vi "Wait on Listener.vi"(8 "error in (no error)":errorcluster, 10 "timeout ms (wait forever: -1)":i32, 11 "TCP slave in":refnum<class "TCP Slave.lvclass">) -> (0 "error out":errorcluster, 1 "timed out?":bool, 2 "connection reference":refnum<data-value>, 3 "TCP slave out":refnum<class "TCP Slave.lvclass">)   [LabVIEW 2020, in "SubVIs.lvlib" / "TCP Slave.lvclass"]
doc: "Wrapper for the wait on listener VI, using the listener stored in the slave and an infinite timeout. When a connection is established, the output class will contain the new connection."
uses:
  <vilib>/Modbus/subvis/Protocol/TCP/TCP Slave/TCP Slave.lvclass
  <vilib>/Modbus/subvis/Protocol/TCP/TCP Slave/TCP Slave.lvclass/TCP Slave.ctl
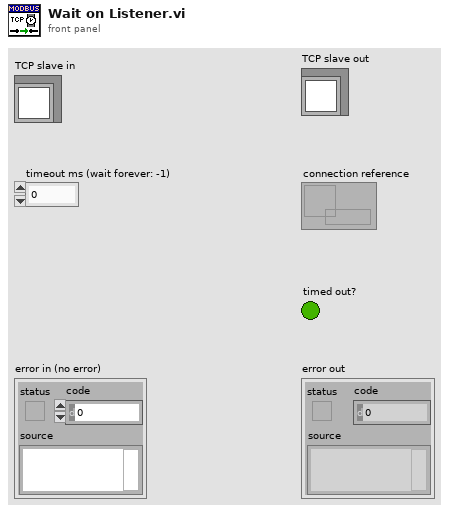
[diagram p1: front panel]
types:
  T1 = cluster{"Connected?":bool, "IP address":string, "connection error":errorcluster}
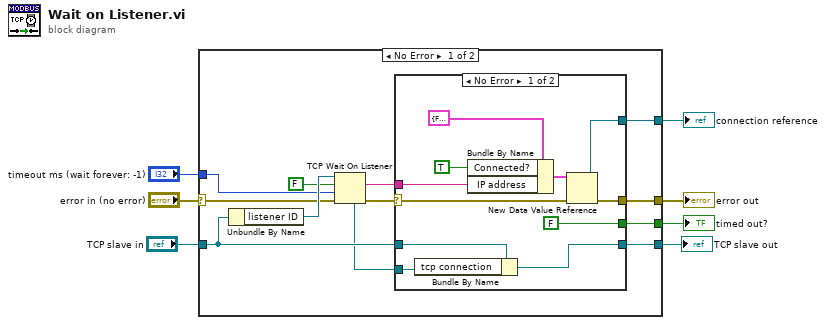
[diagram p0: block diagram]
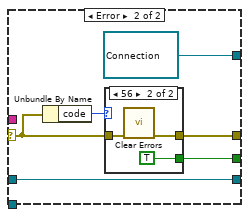
[diagram p2: hidden frame]
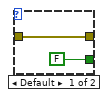
[diagram p3: hidden frame]
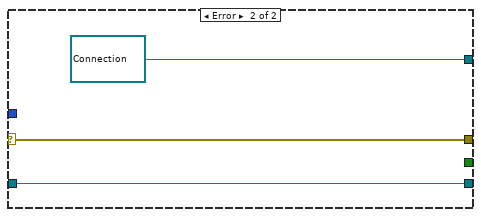
[diagram p4: hidden frame]
diagram:
  n1 = case shown="No Error" "error in (no error)" {
    selector: "error in (no error)" -> [w8 w43]
    tunnel: "TCP slave in" -> [w19 w42]
    tunnel: "timeout ms (wait forever: -1)" -> [w15 _]
    tunnel: [w14 w42] -> w5
    tunnel: [w12 w43] -> w4
    tunnel: [w11 _] -> w3
    tunnel: [w10 refnum<data-value> refnum ("data value reference")] -> w2
    frame No Error {
      n2 = Unbundle By Name(w19) -> ("listener ID"=w18:refnum<k5>)
      n3 = TCP Wait On Listener(8:w8, 9:w15, 10:FALSE ("resolve remote address (T)"), 11:w18) -> (0:w13:errorcluster, 2:w9:string, 4:w17:refnum<k5>)  [unwired: 2 out]
      n4 = case shown="No Error" w13 {
        selector: w13 -> [w26 w35]
        tunnel: w19 -> [w30 w32]
        tunnel: w17 -> [w29 _]
        tunnel: [w27 w32] -> w14
        tunnel: [w20 w34] -> w12
        tunnel: [FALSE w33] -> w11
        tunnel: [w25 refnum<data-value> refnum ("data value reference")] -> w10
        tunnel: w9 -> [w21 _]
        frame No Error {
          n5 = Bundle By Name(cluster=w30, "tcp connection"=w29) -> (w27:refnum<class "TCP Slave.lvclass">)
          n6 = Bundle By Name(cluster=T1 {"Connected?"=FALSE, "IP address"="", "connection error"={"status"=FALSE, "code"=0, "source"=""}} ("Connection"), "Connected?"=TRUE, "IP address"=w21) -> (w23:T1)
          n7 = New Data Value Reference(data value=w23, error in=w26) -> (data value reference=w25:refnum<data-value>, error out=w20:errorcluster)
        }
        frame Error {
          n8 = Unbundle By Name(w35) -> ("code"=w36:i32)
          n9 = case shown="56" w36 {
            tunnel: w35 -> [w38 w41]
            tunnel: [w38 w40] -> w34
            tunnel: [FALSE TRUE] -> w33
            frame Default {
            }
            frame 56 {
              n10 = call <vilib>:"Clear Errors.vi"("error in (no error)"=w41) -> ("error out"=w40:errorcluster)  [unwired: 5 in, 1 out]
            }
          }
        }
      }
    }
    frame Error {
    }
  }
  "error out" <- w4
  "timed out?" <- w3
  "connection reference" <- w2
  "TCP slave out" <- w5
